vi "Tbl_Delete (SubVI).vi"(11 "Table in":refnum<vi>) -> (3 "element":i32)   [LabVIEW 2017]
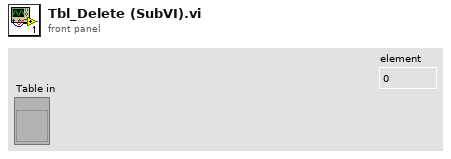
[diagram p1: front panel]
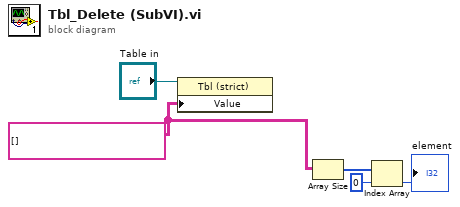
[diagram p0: block diagram]
diagram:
  w4 = string[][] [] ("Protocol")
  n1 = property class="Tbl (strict)"(reference="Table in", "Value"=w4) -> ()  [unwired: 1 in, 2 out]
  n2 = Array Size(array=w4) -> (size(s)=w3:i32[])
  n3 = Index Array(array=w3, index=0) -> (element=→"element":i32)
